vi "new FGGA Serial Data Server & Recordingv4.2.vi"(0 "VISA resource name out":refnum<visa-resource-name>, 11 "error IO":errorcluster) -> ()   [LabVIEW 2014]
uses:
  <vilib>/Platform/TimedLoop/XDataNode/timing_clust.ctl
  <vilib>/Platform/TimedLoop/XDataNode/nitl_modes.ctl
  <vilib>/Platform/TimedLoop/XDataNode/wakeup.ctl
  C:/Program Files (x86)/National Instruments/LabVIEW 2014/examples/Data Communication/Network Streams/Simple Network Streams/support/Network Stream Command.ctl
  <vilib>/Utility/error.llb/whitespace.ctl
  <vilib>/Instr/_visa.llb/VISA Configure Serial Port (Instr).vi
  <vilib>/Utility/tcp.llb/UDP Multicast Write-Only Open.vi
  <vilib>/platform/TimedLoop/XDataNode/XDataNode.xnode
  <vilib>/Platform/TimedLoop/XDataNode/XDNodeRunTimeDep.lvlib
panel:
  out "Unix time":u32
  out "FGGA Pump":bool
  out "Flight Number":string
  out "Stop File Write":bool
  out "Default file name":string
  out "MFC":dbl[](array[numeric])
  out "FGGA restart":bool
  out "V4":bool
  out "V3":bool
  out "V2":bool
  out "V1":bool
  out "error out 2":errorcluster
  out "error out":errorcluster
  in  "MFC_1 SLPM set value":dbl
  out "Value Read":string
  out "status":bool
  in  "VISA resource name":refnum<visa-resource-name>="ASRL3::INSTR"
  in  "timeout (10sec) 2":u32=3000
  in  "Clear Display\nErrors":bool
  out "Data Processing":bool
  out "TCP Binary Packet":string
  out "UDP Time Stamp Offset":i32=1
  out "Data String":string
  out "UDP_ACSII_Out":string
  out "Serial error out":errorcluster
  out "SEPTIC TCP Error Out":errorcluster
  out "TCP packet\nSend To SEPTIC":bool
  out "FISH TCP Error Out":errorcluster
  out "TCP packet\nSend To FISH":bool
  out "UDP_Pack_num":u32
  out "UDP_Out Status":bool
  out "UDP_Out_Error Out":errorcluster
  out "Data Array":string[](array[string])
  out "RAW DATA":string
  in  "stop":bool
  out "Number of times \nRead time out":u32
  out "Loop count":i32
  # "Date"
  # "Time"
  # "CH4_wet_ppm"
  # "1"
  # "CO4_wet_ppm_sd"
  # "H2O_ppm"
  # "3"
  # "H2O_ppm_sd"
  # "CO2_wet_ppm"
  # "5"
  # "CO2_wet_ppm_sd"
  # "CH4_dry_ppm"
  # "CH4_dry_ppm_sd"
  # "CO2_dry_ppm"
  # "CO2_dry_ppm_sd"
  # "cell_pressure_torr"
  # "11"
  # "cell_pressure_torr_sd"
  # "13"
  # "cell_temp_degC"
  # "cell_temp_degC_sdev"
  # "ambient(bench)_temp_degC"
  # "15"
  # "ambient(bench)_temp_dedgC_sd"
  # "17"
  # "RDA_us"
  # "RDA_us_sd"
  # "RDB_us"
  # "19"
  # "RDB_us_sd"
  # "Fitflag"
  # "21"
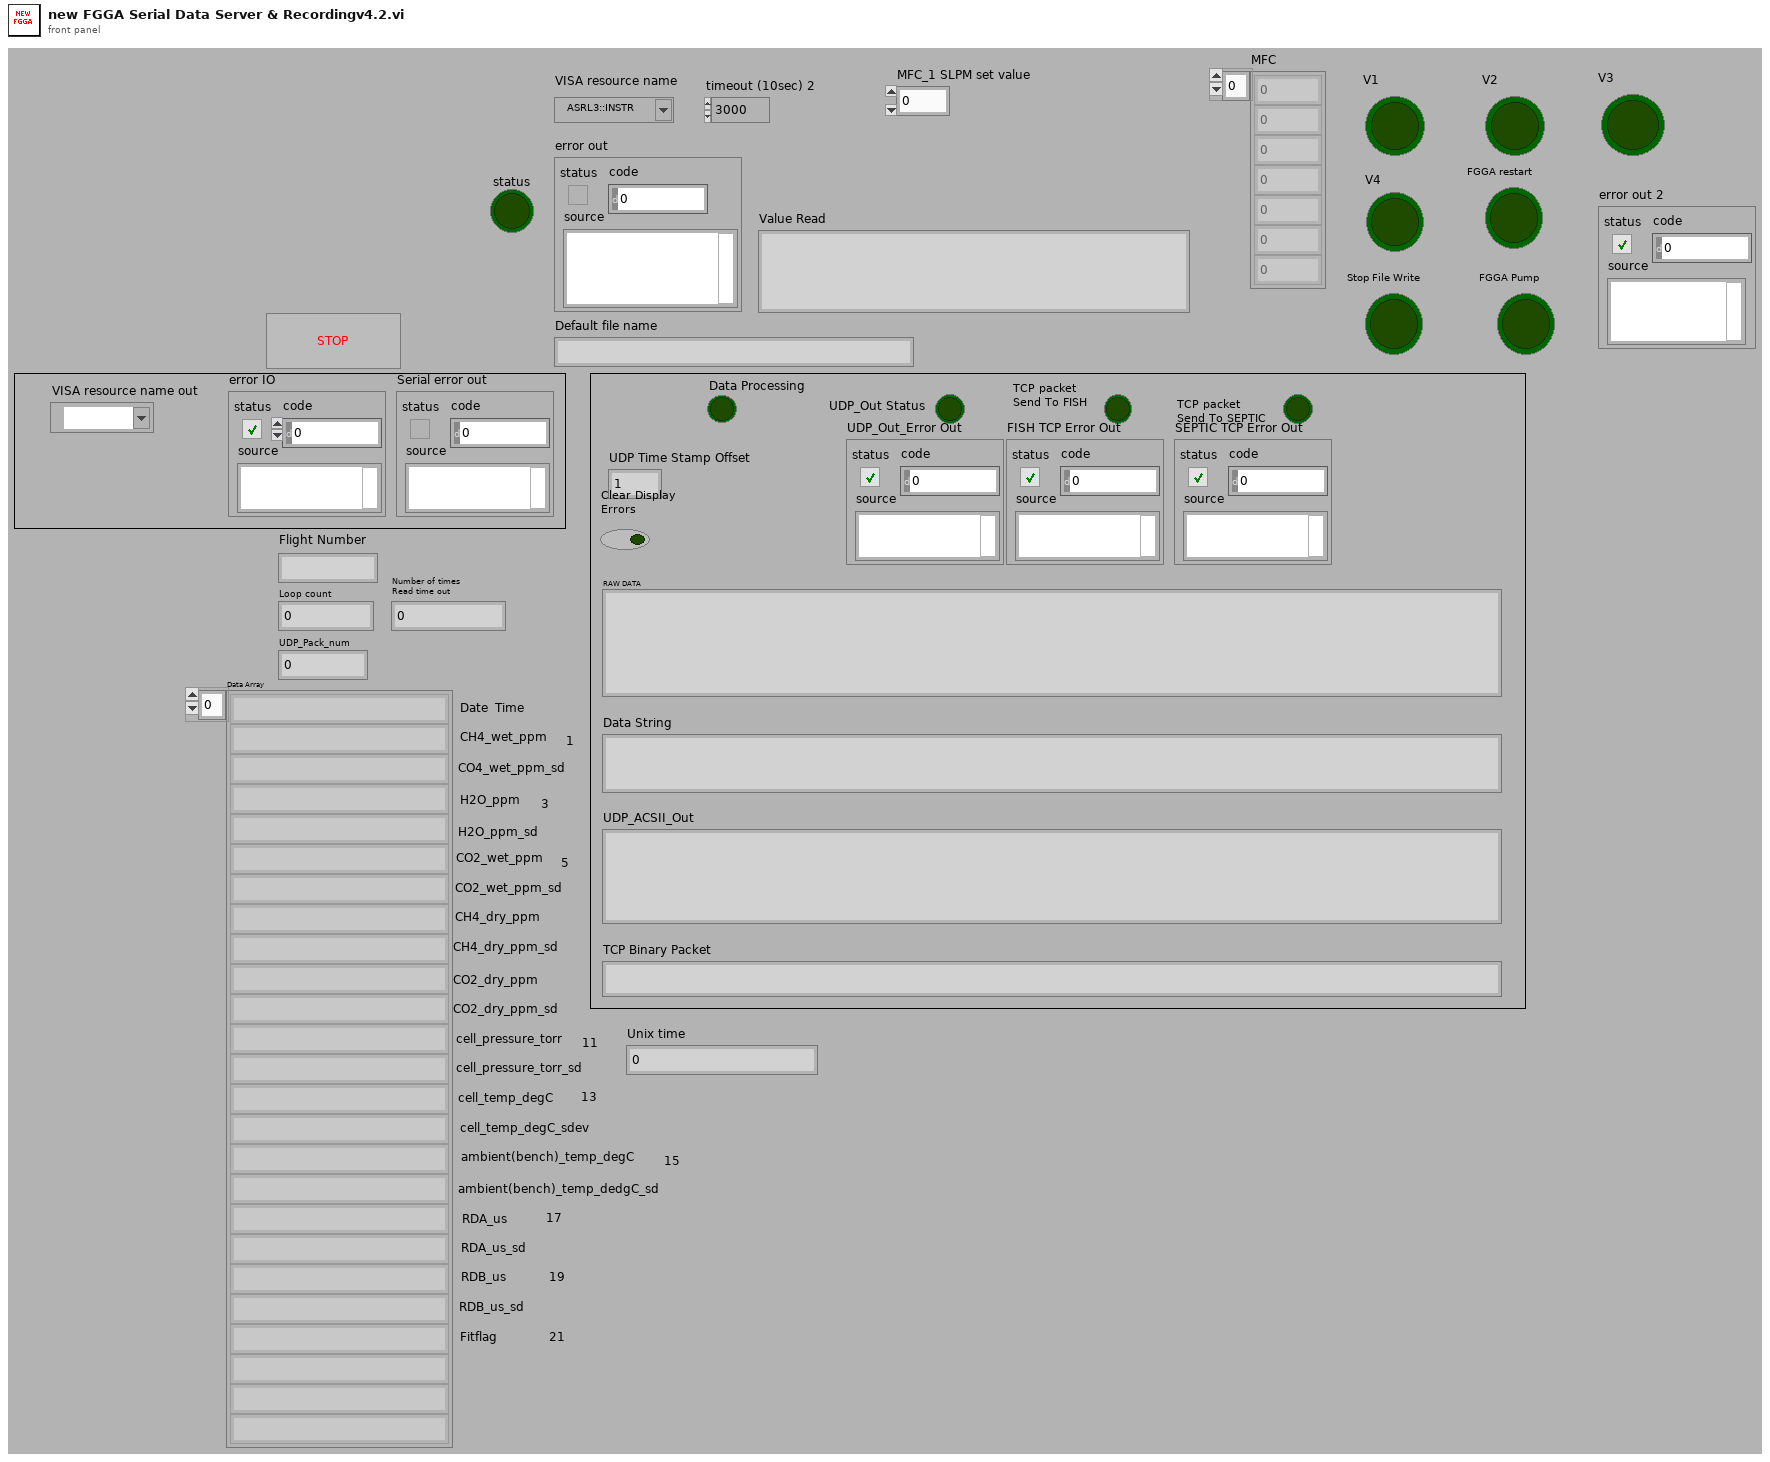
[diagram p1: front panel]
types:
  T1 = typedef "XDNodeRunTimeDep.lvlib/timing_clust.ctl" = cluster{"Expected End [f-1]":u64, "Actual End [f-1]":u64, "Finished Late? [f-1]":bool, "Expected End [i-1]":u64, "Actual End [i-1]":u64, "Finished Late? [i-1]":bool, "Expected Start [i]":u64, "Actual Start [i]":u64, "Expected Start [f]":u64, "Actual Start [f]":u64, "Source Name":string, "Structure Name":string, "Period":i64, "Deadline":i64, "Offset":i64, "Start":i64, "Priority":i32, "Timeout":i32, "Mode":T2, "Wakeup Reason":T3, "Error":errorcluster, "Source Type":string, "Secondary Source Type":string, "Global End Time":u64, "Global Start Time":u64, "Frame Duration":u64, "Iteration Duration":u64, "Assigned CPU":i32, "I/O Scan Engine Mode":u32}
  T2 = typedef "XDNodeRunTimeDep.lvlib/nitl_modes.ctl" = enum32{"No Change", "Process missed periods, maintain original phase", "Discard missed periods, maintain original phase", "Process missed periods, ignore original phase", "Discard missed periods, ignore original phase"}
  T3 = typedef "XDNodeRunTimeDep.lvlib/wakeup.ctl" = enum32{"Normal", "Aborted", "Asynchronous wakeup", "Timing source error", "Timed loop error", "Timeout"}
  T4 = enum16{"open", "replace", "create", "open or create", "replace or create", "replace or create with confirmation"}
  T5 = typedef "Network Stream Command.ctl" = cluster{"Message":string, "Message Data":variant}
  T6 = typedef "whitespace.ctl" = u16
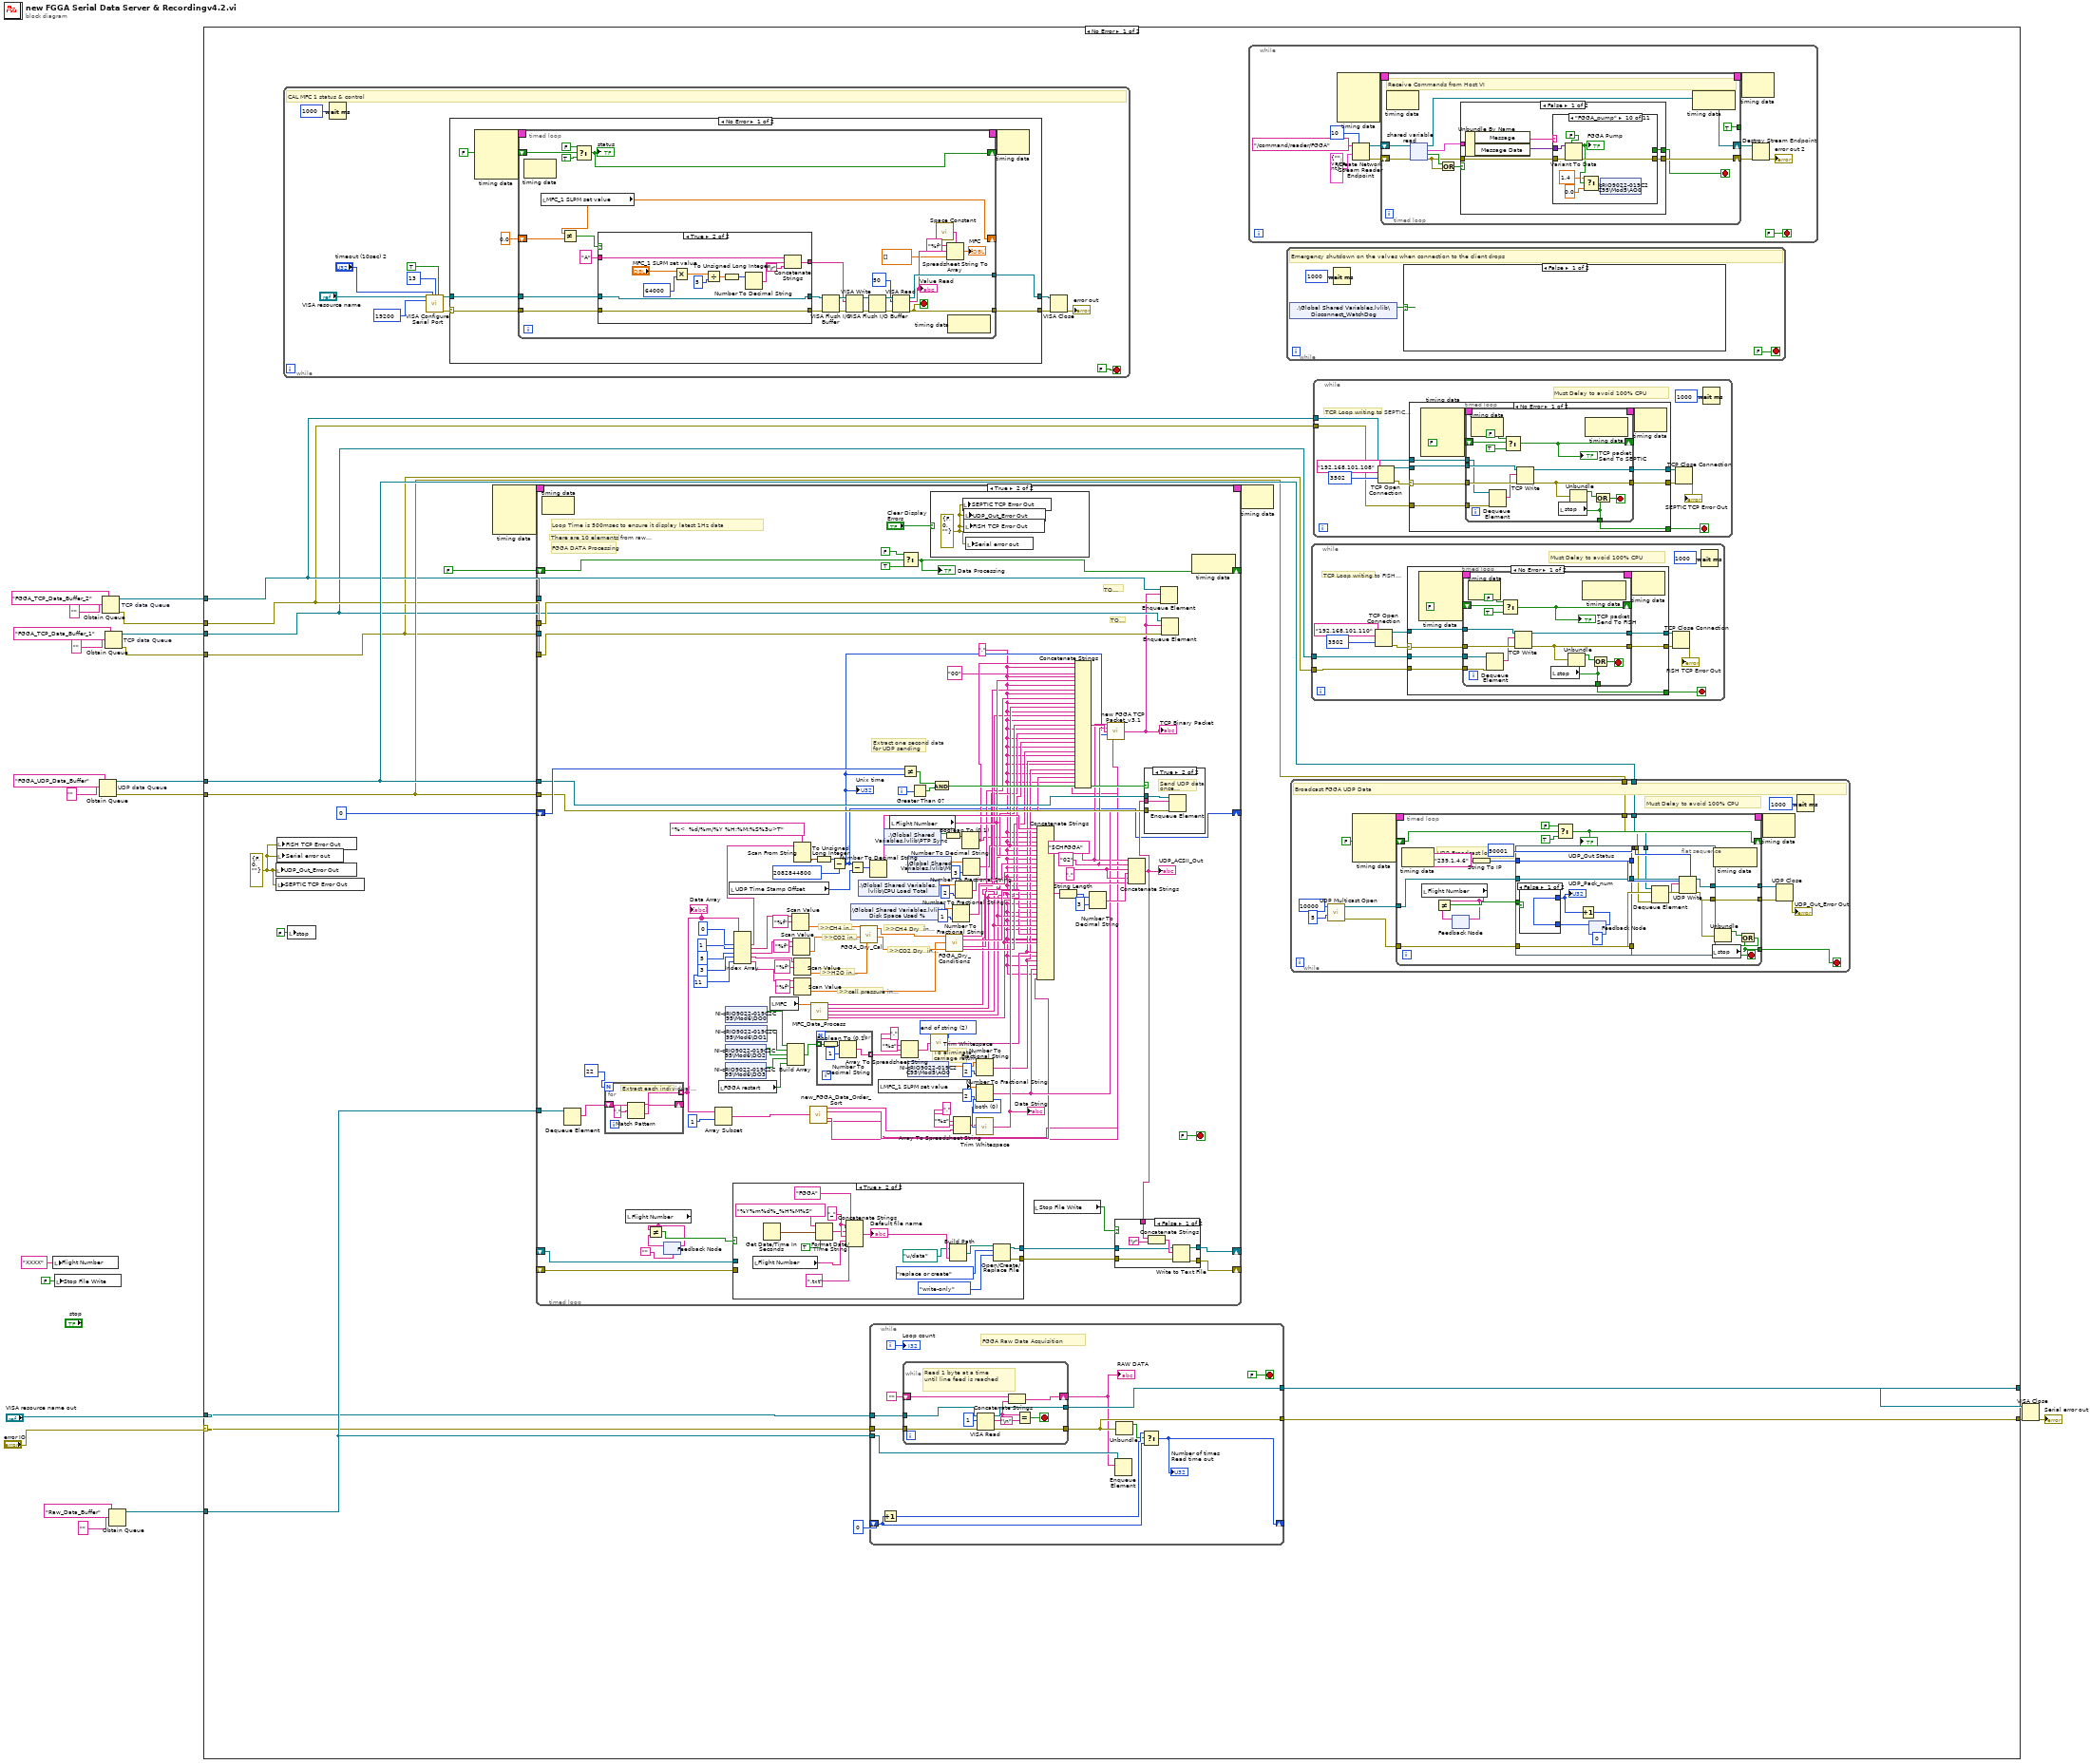
[diagram p0: block diagram]
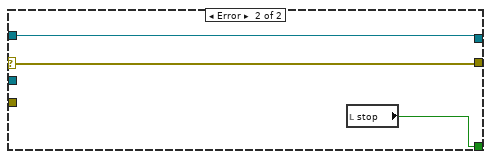
[diagram p2: hidden frame]
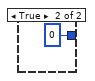
[diagram p3: hidden frame]
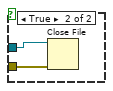
[diagram p5: hidden frame]
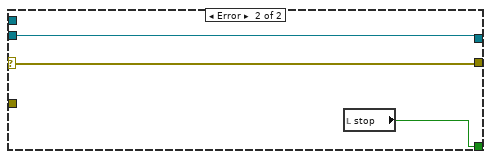
[diagram p8: hidden frame]
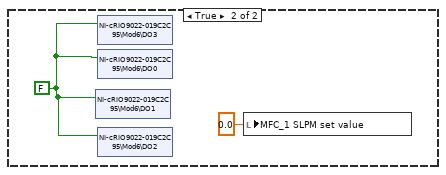
[diagram p9: hidden frame]
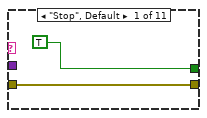
[diagram p10: hidden frame]
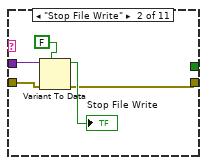
[diagram p11: hidden frame]
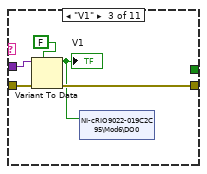
[diagram p12: hidden frame]
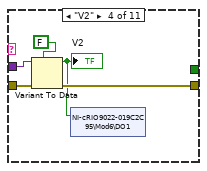
[diagram p13: hidden frame]
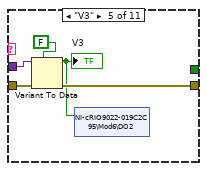
[diagram p14: hidden frame]
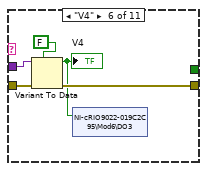
[diagram p15: hidden frame]
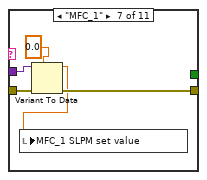
[diagram p16: hidden frame]
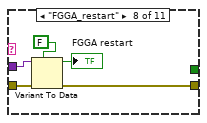
[diagram p17: hidden frame]
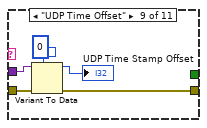
[diagram p18: hidden frame]
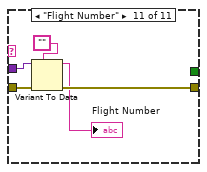
[diagram p19: hidden frame]
diagram:
  n1 = local write "Flight Number"("XXXX" ("Flight Number")) -> ()
  n2 = local write "Stop File Write"(FALSE ("Stop File Write")) -> ()
  n3 = Obtain Queue "UDP data Queue"(name (unnamed)="FGGA_UDP_Data_Buffer", element data type="") -> (queue out=w14:refnum<queue>, error out=w13:errorcluster)  [unwired: 3 in, 1 out]
  n4 = Obtain Queue "TCP data Queue"(name (unnamed)="FGGA_TCP_Data_Buffer_2", element data type="") -> (queue out=w8:refnum<queue>, error out=w7:errorcluster)  [unwired: 3 in, 1 out]
  n5 = Obtain Queue "TCP data Queue"(name (unnamed)="FGGA_TCP_Data_Buffer_1", element data type="") -> (queue out=w6:refnum<queue>, error out=w5:errorcluster)  [unwired: 3 in, 1 out]
  n6 = Obtain Queue(name (unnamed)="Raw_Data_Buffer", element data type="") -> (queue out=w20:refnum<queue>)  [unwired: 3 in, 2 out]
  n7 = case shown="No Error" "error IO" {
    selector: "error IO" -> [w27 w536]
    tunnel: "VISA resource name out" -> [w28 w537]
    tunnel: [w39 w537] -> w17
    tunnel: [w40 w536] -> w18
    tunnel: w20 -> [w38 _]
    tunnel: w14 -> [w36 _]
    tunnel: w13 -> [w35 _]
    tunnel: w8 -> [w34 _]
    tunnel: w7 -> [w33 _]
    tunnel: w6 -> [w32 _]
    tunnel: w5 -> [w31 _]
    frame No Error {
      w23 = errorcluster {"status"=FALSE, "code"=0, "source"=""} ("UDP Error Out")
      n8 = local write "UDP_Out_Error Out"(w23) -> ()
      n9 = local write "SEPTIC TCP Error Out"(w23) -> ()
      n10 = local write "FISH TCP Error Out"(w23) -> ()
      n11 = local write "Serial error out"(w23) -> ()
      n12 = while {
        stop <- FALSE stop-if-true
        # "CAL MFC 1 status & control"
        n13 = Wait (ms)(milliseconds to wait=u32 1000) -> ()  [unwired: 1 out]
        n14 = call-poly "VISA Configure Serial Port"("VISA resource name"="VISA resource name", "timeout (10sec)"="timeout (10sec) 2", "termination char\n(0xA = '\\n' = LF)"=u8 13 ("termination char\n(0xA = '\\n' = LF)"), "Enable Termination\nChar (T)"=TRUE ("Enable Termination\nChar (T)"), "baud rate (9600)"=u32 19200) -> ("VISA resource name out"=w477:refnum<visa-resource-name>, "error out"=w473:errorcluster)  [unwired: 9 in]
        n15 = case shown="No Error" w473 {
          selector: w473 -> [w484 w534]
          tunnel: w477 -> [w485 w535]
          tunnel: [w483 w535] -> w476
          tunnel: [w482 w534] -> w475
          frame No Error {
            n16 = node-c288() -> (w480:T1)  [unwired: 4 in]
            n17 = timed-loop {
              tunnel: w485 -> [w508]
              tunnel: w484 -> [w506]
              tunnel: [w499] -> w483
              tunnel: [w494] -> w482
              shift-right: [w495] -> _
              shift-left: FALSE -> [w498]
              timing: w480 -> [_]
              timing-out: [_] -> w479
              shift-right: [w486] -> _
              shift-left: 0.0 -> [w488]
              stop <- w494 stop-if-true
              n18 = node-c288() -> ()  [unwired: 1 in, 1 out]
              n19 = local read "MFC_1 SLPM set value"() -> (w486:dbl)
              n20 = Not Equal?(x=w486, y=w488) -> (x != y?=w487:bool)
              n21 = Select(t=FALSE, s=w498, f=TRUE) -> (s? t:f=w495:bool)
              "status" <- w495
              n22 = case shown="True" w487 {
                tunnel: w508 -> [w516 w531]
                tunnel: [w516 w531] -> w507
                tunnel: w506 -> [w515 w530]
                tunnel: [w515 w530] -> w505
                tunnel: "A" -> [w519 w523]
                tunnel: [w517 w520] -> w503
                frame False {
                  n23 = Concatenate Strings(w519, "\r") -> (w517:string)
                }
                frame True {
                  n24 = Multiply(x="MFC_1 SLPM set value", y=u32 64000) -> (x*y=w527:dbl)
                  n25 = Divide(x=w527, y=u32 5) -> (x/y=w525:dbl)
                  n26 = To Unsigned Long Integer(number=w525) -> (unsigned 32bit integer=w524:u32)
                  n27 = Number To Decimal String(number=w524) -> (decimal integer string=w522:string)  [unwired: 1 in]
                  n28 = Concatenate Strings(w523, w522, "\r") -> (w520:string)
                }
              }
              n29 = VISA Flush I/O Buffer(VISA resource name=w507, error in (no error)=w505) -> (VISA resource name out=w510:refnum<visa-resource-name>, error out=w509:errorcluster)  [unwired: 1 in]
              n30 = VISA Write(VISA resource name=w510, write buffer=w503, error in (no error)=w509) -> (VISA resource name out=w502:refnum<visa-resource-name>, error out=w501:errorcluster)  [unwired: 1 out]
              n31 = VISA Flush I/O Buffer(VISA resource name=w502, error in (no error)=w501) -> (VISA resource name out=w512:refnum<visa-resource-name>, error out=w511:errorcluster)  [unwired: 1 in]
              n32 = VISA Read(VISA resource name=w512, byte count=u32 50, error in (no error)=w511) -> (VISA resource name out=w499:refnum<visa-resource-name>, read buffer=w493:string, error out=w494:errorcluster)  [unwired: 1 out]
              "Value Read" <- w493
              n33 = call <vilib>:"Space Constant.vi"() -> ("String"=w492:string)
              n34 = Spreadsheet String To Array(delimiter (Tab)=w492, format string="%f", spreadsheet string=w493, array type (2D Dbl)=dbl[] []) -> (array=→"MFC":dbl[])
              n35 = node-c288() -> ()  [unwired: 1 in, 1 out]
            }
            n36 = node-c288(w479) -> ()  [unwired: 1 out]
          }
          frame Error {
          }
        }
        n37 = VISA Close(VISA resource name=w476, error in (no error)=w475) -> (error out=→"error out":errorcluster)
      }
      n38 = local write "stop"(FALSE ("stop")) -> ()
      n39 = node-c288() -> (w25:T1)  [unwired: 4 in]
      n40 = timed-loop {
        timing: w25 -> [_]
        timing-out: [_] -> w24
        tunnel: w38 -> [w265]
        tunnel: w36 -> [w230]
        tunnel: w35 -> [w229]
        shift-right: [w155] -> _
        shift-left: u32 0 -> [w233]
        tunnel: w34 -> [w228]
        tunnel: w33 -> [w227]
        tunnel: w32 -> [w226]
        tunnel: w31 -> [w225]
        shift-right: [w221] -> _
        shift-left: FALSE -> [w224]
        shift-right: [w210] -> _
        shift-left: _ -> [w202]
        shift-right: [w200] -> _
        shift-left: _ -> [w201]
        i -> [w232]
        stop <- FALSE stop-if-true
        w174 = T6 2 items=["both", "start of string", "end of string"] ("location (both)")
        w148 = ","
        w251 = T6 0 items=["both", "start of string", "end of string"] ("location (both)")
        w259 = ","
        w156 = "02"
        w157 = "$CHFGGA"
        # "To eliminate\ncarriage return"
        # ">>cell pressure in torr>>"
        # "There are 10 elements from raw packet"
        # "TO SEPTIC"
        # "TO FISH"
        # "Extract one second data\nfor UDP sending"
        # ">>CO2 Dry  in ppm>>"
        # ">>CH4 Dry  in ppb>>"
        # ">>H2O in ppm>>"
        # ">>CO2 in ppm>>"
        # ">>CH4 in ppm>>"
        # "Loop Time is 500msec to ensure it display latest 1Hz data"
        # "FGGA DATA Processing"
        n41 = node-c288() -> ()  [unwired: 1 in, 1 out]
        n42 = Dequeue Element(queue=w265) -> (element=w220:string)  [unwired: 2 in, 3 out]
        n43 = for {
          N: 22 -> [_]
          shift-right: [w302] -> _
          shift-left: w220 -> [w300]
          tunnel: [w301] -> w256 mode=indexing
          # "Extract each individual param"
          n44 = Match Pattern(string=w300, regular expression=",") -> (before substring=w301:string, after substring=w302:string)  [unwired: 1 in, 2 out]
        }
        "Data Array" <- w256
        n45 = local read "Flight Number"() -> (w199:string)
        n46 = feedback #1("" ("Flight Number")) -> (w207:string)
        n47 = Not Equal?(x=w199, y=w207) -> (x != y?=w205:bool)
        n48 = feedback-in #1(w199) -> ()
        n49 = Array Subset(array=w256, index=1) -> (w146:string[])  [unwired: 1 in]
        n50 = local read "FGGA restart"() -> (w184:bool)
        n51 = shared-variable "NI-cRIO9022-019C2C95\\Mod6\\DO2"() -> (w190:bool)  [unwired: 1 in, 1 out]
        n52 = shared-variable "NI-cRIO9022-019C2C95\\Mod6\\DO3"() -> (w189:bool)  [unwired: 1 in, 1 out]
        n53 = shared-variable "NI-cRIO9022-019C2C95\\Mod6\\DO0"() -> (w192:bool)  [unwired: 1 in, 1 out]
        n54 = shared-variable "NI-cRIO9022-019C2C95\\Mod6\\DO1"() -> (w191:bool)  [unwired: 1 in, 1 out]
        n55 = local read "UDP Time Stamp Offset"() -> (w173:i32)
        n56 = case shown="True" w205 {
          tunnel: [w271 w273] -> w204
          tunnel: [w270 w272] -> w203
          tunnel: w202 -> [w271 _]
          tunnel: w201 -> [w270 _]
          frame False {
          }
          frame True {
            w279 = "_" ("string")
            n57 = local read "Flight Number"() -> (w286:string)
            n58 = Get Date/Time In Seconds() -> (seconds since 1Jan1904=w274:timestamp)
            n59 = Format Date/Time String(time format string (%c)="%Y%m%d%_%H%M%S", seconds (now)=w274, UTC format=TRUE) -> (date/time string=w276:string)
            n60 = Concatenate Strings("FGGA" ("string"), w279, w276, w279, w286, ".txt" ("string")) -> (w281:string)
            "Default file name" <- w281
            n61 = Build Path(base path=path "u:/data", name or relative path=w281) -> (appended path=w285:path)
            n62 = Open/Create/Replace File(file path (use dialog)=w285, operation (0:open)=T4."replace or create", access (0:read/write)=enum16{"read/write", "read-only", "write-only"}."write-only") -> (refnum out=w273:refnum<file>, error out=w272:errorcluster)  [unwired: 3 in, 1 out]
          }
        }
        n63 = Index Array(array=w256, index #1=0 ("index"), index #2=1 ("index"), index #3=5 ("index"), index #4=3 ("index"), index #5=11 ("index")) -> (element #1=w149:string, element #2=w154:string, element #3=w153:string, element #4=w152:string, element #5=w151:string)
        n64 = local read "MFC"() -> (w211:dbl[])
        n65 = Build Array(w192, w191, w190, w189, w184) -> (w188:bool[])
        n66 = Scan Value(string=w154, format string="%f") -> (value=w242:dbl)  [unwired: 1 in, 1 out]
        n67 = Scan Value(string=w153, format string="%f") -> (value=w241:dbl)  [unwired: 1 in, 1 out]
        n68 = Scan From String(format string="%<  %d/%m/%Y %H:%M:%S%3u>T", input string=w149) -> (output 1=w238:timestamp)  [unwired: 3 in, 3 out]
        n69 = Scan Value(string=w152, format string="%f") -> (value=w212:dbl)  [unwired: 1 in, 1 out]
        n70 = Scan Value(string=w151, format string="%f") -> (value=w213:dbl)  [unwired: 1 in, 1 out]
        n71 = call "new_FGGA_Data_Order_Sort.vi"("Data In"=w146) -> ("UDP Data Out"=w145:string[], "UDP Ambient(bench)_temp"=w144:string, "TCP Data Out"=w143:string[], "TCP Ambient(bench)_temp"=w142:string)  [unwired: 11 in]
        n72 = call "MFC_Data_Process.vi"("MFC"=w211) -> ("MFC Absolute Pressure"=w168:string, "MFC Temperature"=w167:string, "MFC Volumetric Flow"=w166:string, "MFC Mass Flow"=w165:string, "MFC Set Point"=w164:string)  [unwired: 10 in]
        n73 = To Unsigned Long Integer(number=w238) -> (unsigned 32bit integer=w239:u32)
        n74 = for {
          tunnel: w188 -> [w268] mode=indexing
          tunnel: [w267] -> w185 mode=indexing
          n75 = Boolean To (0,1)(Boolean=w268) -> (0, 1=w269:i16)
          n76 = Number To Decimal String(number=w269, width (-)=i16 1) -> (decimal integer string=w267:string)
        }
        n77 = Subtract(x=w239, y=u32 2082844800) -> (x-y=w155:u32)
        "Unix time" <- w155
        n78 = Subtract(x=w155, y=w173) -> (x-y=w236:u32)
        n79 = shared-variable ".\\Global Shared Variables.lvlib\\Disk Space Used %"() -> (w177:dbl)  [unwired: 1 in, 1 out]
        n80 = shared-variable ".\\Global Shared Variables.lvlib\\CPU Load Total"() -> (w198:dbl)  [unwired: 1 in, 1 out]
        n81 = call "FGGA_Dry_Cal.vi"("H2O"=w212, "CO2_Wet"=w241, "CH4_Wet"=w242) -> ("CO2_Dry"=w215:dbl, "CH4_Dry"=w217:dbl)  [unwired: 7 in]
        n82 = Number To Decimal String(number=w236) -> (decimal integer string=w237:string)  [unwired: 1 in]
        n83 = local read "MFC_1 SLPM set value"() -> (w180:dbl)
        n84 = shared-variable ".\\Global Shared Variables.lvlib\\PTP Sync"() -> (w193:bool)  [unwired: 1 in, 1 out]
        n85 = local read "Flight Number"() -> (w172:string)
        n86 = Array To Spreadsheet String(delimiter (Tab)=",", array=w185, 3:"%s" ("format string")) -> (spreadsheet string=w175:string)
        n87 = Select(t=FALSE, s=w224, f=TRUE) -> (s? t:f=w221:bool)
        "Data Processing" <- w221
        n88 = Not Equal?(x=w233, y=w155) -> (x != y?=w234:bool)
        n89 = shared-variable ".\\Global Shared Variables.lvlib\\MFM"() -> (w196:dbl)  [unwired: 1 in, 1 out]
        n90 = shared-variable "NI-cRIO9022-019C2C95\\Mod5\\AO0"() -> (w182:dbl)  [unwired: 1 in, 1 out]
        n91 = Greater Than 0?(x=w232) -> (x > 0?=w235:bool)
        n92 = case shown="True" "Clear Display\nErrors" {
          frame False {
          }
          frame True {
            w296 = errorcluster {"status"=FALSE, "code"=0, "source"=""} ("UDP Error Out")
            n93 = local write "SEPTIC TCP Error Out"(w296) -> ()
            n94 = local write "UDP_Out_Error Out"(w296) -> ()
            n95 = local write "FISH TCP Error Out"(w296) -> ()
            n96 = local write "Serial error out"(w296) -> ()
          }
        }
        n97 = call <vilib>:"Trim Whitespace.vi"("string"=w175, "location (both)"=w174) -> ("trimmed string"=w163:string)
        n98 = Compound Arithmetic op=AND(w234, w235) -> (w231:bool)
        n99 = Boolean To (0,1)(Boolean=w193) -> (0, 1=w194:i16)
        n100 = call "FGGA_Dry_Conditions.vi"("CH4_Dry"=w217, "Pressure"=w213, "CO2_Dry"=w215) -> ("CH4_Dry_TCP"=w171:string, "CH4_Dry_UDP"=w219:string, "CO2_Dry_TCP"=w170:string, "CO2_Dry_UDP"=w218:string)  [unwired: 9 in]
        n101 = Number To Fractional String(number=w177, precision (6)=i16 1) -> (F-format string=w176:string)  [unwired: 2 in]
        n102 = Array To Spreadsheet String(delimiter (Tab)=",", array=w145, 3:"%s" ("format string")) -> (spreadsheet string=w250:string)
        n103 = Number To Fractional String(number=w198, precision (6)=i16 2) -> (F-format string=w179:string)  [unwired: 2 in]
        n104 = Number To Decimal String(number=w194) -> (decimal integer string=w159:string)  [unwired: 1 in]
        n105 = Number To Fractional String(number=w196, precision (6)=i16 3) -> (F-format string=w169:string)  [unwired: 2 in]
        n106 = Number To Fractional String(number=w182, precision (6)=i16 2) -> (F-format string=w162:string)  [unwired: 2 in]
        n107 = Number To Fractional String(number=w180, precision (6)=i16 2) -> (F-format string=w161:string)  [unwired: 2 in]
        n108 = call <vilib>:"Trim Whitespace.vi"("string"=w250, "location (both)"=w251) -> ("trimmed string"=w249:string)
        "Data String" <- w249
        n109 = local read "Stop File Write"() -> (w208:bool)
        n110 = Concatenate Strings(w237, w148, w159, w148, w169, w148, w172, w148, w179, w148, w176, w148, w249, w148, w219, w148, w218, w148, w168, w148, w167, w148, w166, w148, w165, w148, w164, w148, w163, w148, w162, w148, w161, w148, w144) -> (w258:string)
        n111 = String Length(string=w258) -> (length=w262:i32)
        n112 = Concatenate Strings(w159, w148, "00", w148, w172, w148, w171, w148, w170, w148, w169, w148, w168, w148, w167, w148, w166, w148, w165, w148, w164, w148, w163, w148, w162, w148, w161, w148, w142) -> (w160:string)
        n113 = Number To Decimal String(number=w262, width (-)=i16 3) -> (decimal integer string=w260:string)
        n114 = call "new FGGA TCP Packet_v3.1.vi"("ID"=w157, "Version"=w156, "TCP Packet In"=w160, "utc_time"=w155, "Data Array"=w143) -> ("TCP Binary Packet"=w147:string)  [unwired: 10 in]
        "TCP Binary Packet" <- w147
        n115 = Concatenate Strings(w157, w156, w259, w260, w259, w258) -> (w209:string)
        "UDP_ACSII_Out" <- w209
        n116 = case shown="False" w208 {
          tunnel: w209 -> [w293 _]
          tunnel: [w290 _] -> w210
          tunnel: w204 -> [w289 w295]
          tunnel: w203 -> [w288 w294]
          tunnel: [w287 _] -> w200
          frame False {
            n117 = Concatenate Strings(w293, "\r") -> (w291:string)
            n118 = Write to Text File(file (use dialog)=w289, text=w291, error in=w288) -> (refnum out=w290:refnum<file>, error out=w287:errorcluster)  [unwired: 2 out]
          }
          frame True {
            n119 = Close File(refnum=w295, error in=w294) -> ()  [unwired: 2 out]
          }
        }
        n120 = case shown="True" w231 {
          tunnel: w209 -> [_ w299]
          tunnel: w230 -> [_ w298]
          tunnel: w229 -> [_ w297]
          frame False {
          }
          frame True {
            # "Send UDP data once\na second"
            n121 = Enqueue Element(queue=w298, element=w299, error in (no error)=w297) -> ()  [unwired: 1 in, 3 out]
          }
        }
        n122 = Enqueue Element(queue=w228, element=w147, error in (no error)=w227) -> ()  [unwired: 1 in, 3 out]
        n123 = Enqueue Element(queue=w226, element=w147, error in (no error)=w225) -> ()  [unwired: 1 in, 3 out]
        n124 = node-c288() -> ()  [unwired: 1 in, 1 out]
      }
      n125 = while {
        tunnel: w28 -> [w362]
        tunnel: w27 -> [w361]
        tunnel: [w360] -> w40
        shift-right: [w356] -> _
        shift-left: u32 0 -> [w357]
        tunnel: [w359] -> w39
        tunnel: w38 -> [w353]
        i -> [w358]
        stop <- FALSE stop-if-true
        # "FGGA Raw Data Acquisition"
        n126 = Increment(x=w357) -> (x+1=w355:u32)
        n127 = while {
          tunnel: [w372] -> w359
          tunnel: [w371] -> w360
          tunnel: w362 -> [w370]
          tunnel: w361 -> [w369]
          shift-right: [w367] -> w352
          shift-left: "" -> [w368]
          stop <- w364 stop-if-true
          # "Read 1 byte at a time \nuntil line feed is reached"
          n128 = VISA Read(VISA resource name=w370, byte count=u32 1, error in (no error)=w369) -> (VISA resource name out=w372:refnum<visa-resource-name>, read buffer=w366:string, error out=w371:errorcluster)  [unwired: 1 out]
          n129 = Concatenate Strings(w368, w366) -> (w367:string)
          n130 = Equal?(x=w366, y="\n") -> (x = y?=w364:bool)
        }
        "RAW DATA" <- w352
        n131 = Enqueue Element(queue=w353, element=w352) -> ()  [unwired: 2 in, 3 out]
        n132 = Unbundle(w360) -> ("status"=w351:bool)  [unwired: 2 out]
        n133 = Select(t=w355, s=w351, f=w357) -> (s? t:f=w356:u32)
        "Number of times \nRead time out" <- w356
        "Loop count" <- w358
      }
      n134 = node-c288(w24) -> ()  [unwired: 1 out]
      n135 = while {
        stop <- FALSE stop-if-true
        n136 = node-c288() -> (w379:T1)  [unwired: 4 in]
        n137 = Create Network Stream Reader Endpoint(7:10 ("reader buffer size"), 9:T5 {"Message"="", "Message Data"=variant} ("Message Cluster"), 11:"/command/reader/FGGA" ("reader url")) -> (0:w384:errorcluster, 3:w385:refnum<k21>)  [unwired: 4 in]
        n138 = timed-loop "Host->Target Command Reader" {
          shift-right: [w395] -> w382
          shift-left: w384 -> [w398]
          shift-right: [w396] -> w381
          shift-left: w385 -> [w397]
          tunnel: [TRUE] -> _
          timing: w379 -> [_]
          timing-out: [_] -> w378
          stop <- w389 stop-if-true
          # "Receive Commands from Host VI"
          n139 = node-c288() -> ()  [unwired: 1 in, 1 out]
          n140 = shared-variable-read(w397, w398) -> (w396:refnum<k21>, w391:errorcluster, w393:bool, w394:T5)  [unwired: 1 in]
          n141 = Or(x=w393, y=w391) -> (x .or. y?=w392:bool)
          n142 = case shown="False" w392 {
            selector: w392 -> [_ w462]
            tunnel: w391 -> [w406 w463]
            tunnel: [w405 w463] -> w395
            tunnel: w394 -> [w403 _]
            tunnel: [w404 w462] -> w389
            frame False {
              n143 = Unbundle By Name(w403) -> ("Message"=w402:string, "Message Data"=w401:variant)
              n144 = case shown="\"FGGA_pump\"" w402 {
                tunnel: w406 -> [w408 w413 w418 w423 w428 w433 w438 w443 w448 w456 w461]
                tunnel: [w408 w409 w417 w422 w427 w432 w437 w442 w447 w455 w460] -> w405
                tunnel: w401 -> [_ w412 w416 w421 w426 w431 w436 w441 w446 w454 w459]
                tunnel: [TRUE _ _ _ _ _ _ _ _ _ _] -> w404
                frame "Stop", Default {
                }
                frame "Stop File Write" {
                  n145 = Variant To Data(error in=w413, type=FALSE, Variant=w412) -> (data=→"Stop File Write":bool, error out=w409:errorcluster)
                }
                frame "V1" {
                  n146 = Variant To Data(error in=w418, type=FALSE, Variant=w416) -> (data=w414:bool, error out=w417:errorcluster)
                  "V1" <- w414
                  n147 = shared-variable "NI-cRIO9022-019C2C95\\Mod6\\DO0"(w414) -> ()  [unwired: 1 in, 1 out]
                }
                frame "V2" {
                  n148 = Variant To Data(error in=w423, type=FALSE, Variant=w421) -> (data=w419:bool, error out=w422:errorcluster)
                  "V2" <- w419
                  n149 = shared-variable "NI-cRIO9022-019C2C95\\Mod6\\DO1"(w419) -> ()  [unwired: 1 in, 1 out]
                }
                frame "V3" {
                  n150 = Variant To Data(error in=w428, type=FALSE, Variant=w426) -> (data=w424:bool, error out=w427:errorcluster)
                  "V3" <- w424
                  n151 = shared-variable "NI-cRIO9022-019C2C95\\Mod6\\DO2"(w424) -> ()  [unwired: 1 in, 1 out]
                }
                frame "V4" {
                  n152 = Variant To Data(error in=w433, type=FALSE, Variant=w431) -> (data=w429:bool, error out=w432:errorcluster)
                  "V4" <- w429
                  n153 = shared-variable "NI-cRIO9022-019C2C95\\Mod6\\DO3"(w429) -> ()  [unwired: 1 in, 1 out]
                }
                frame "MFC_1" {
                  n154 = Variant To Data(error in=w438, type=0.0, Variant=w436) -> (data=w434:dbl, error out=w437:errorcluster)
                  n155 = local write "MFC_1 SLPM set value"(w434) -> ()
                }
                frame "FGGA_restart" {
                  n156 = Variant To Data(error in=w443, type=FALSE, Variant=w441) -> (data=→"FGGA restart":bool, error out=w442:errorcluster)
                }
                frame "UDP Time Offset" {
                  n157 = Variant To Data(error in=w448, type=0, Variant=w446) -> (data=→"UDP Time Stamp Offset":i32, error out=w447:errorcluster)
                }
                frame "FGGA_pump" {
                  n158 = Variant To Data(error in=w456, type=FALSE, Variant=w454) -> (data=w451:bool, error out=w455:errorcluster)
                  "FGGA Pump" <- w451
                  n159 = Select(t=1.4 ("f"), s=w451, f=0.0 ("t")) -> (s? t:f=w452:dbl)
                  n160 = shared-variable "NI-cRIO9022-019C2C95\\Mod5\\AO0"(w452) -> ()  [unwired: 1 in, 1 out]
                }
                frame "Flight Number" {
                  n161 = Variant To Data(error in=w461, type="", Variant=w459) -> (data=→"Flight Number":string, error out=w460:errorcluster)
                }
              }
            }
            frame True {
            }
          }
          n162 = node-c288() -> ()  [unwired: 1 in, 1 out]
        }
        n163 = node-c288(w378) -> ()  [unwired: 1 out]
        n164 = Destroy Stream Endpoint(8:w382, 11:w381) -> (0:→"error out 2":errorcluster)
      }
      n165 = while {
        stop <- FALSE stop-if-true
        # "Emergency shutdown on the valves when connection to the client drops"
        n166 = shared-variable ".\\Global Shared Variables.lvlib\\Disconnect_WatchDog"() -> (w373:bool)  [unwired: 1 in, 1 out]
        n167 = Wait (ms)(milliseconds to wait=u32 1000) -> ()  [unwired: 1 out]
        n168 = case shown="False" w373 {
          frame False {
          }
          frame True {
            w377 = FALSE
            n169 = shared-variable "NI-cRIO9022-019C2C95\\Mod6\\DO1"(w377) -> ()  [unwired: 1 in, 1 out]
            n170 = shared-variable "NI-cRIO9022-019C2C95\\Mod6\\DO3"(w377) -> ()  [unwired: 1 in, 1 out]
            n171 = shared-variable "NI-cRIO9022-019C2C95\\Mod6\\DO0"(w377) -> ()  [unwired: 1 in, 1 out]
            n172 = shared-variable "NI-cRIO9022-019C2C95\\Mod6\\DO2"(w377) -> ()  [unwired: 1 in, 1 out]
            n173 = local write "MFC_1 SLPM set value"(0.0 ("MFC_1 SLPM set value")) -> ()
          }
        }
      }
      n174 = while {
        tunnel: w36 -> [w85]
        tunnel: w35 -> [w84]
        stop <- w86 stop-if-true
        # "Must Delay to avoid 100% CPU"
        # "Broadcast FGGA UDP Data"
        n175 = call-poly <vilib>:"UDP Multicast Open.vi"("time-to-live (1)"=u16 5, "port"=u16 10000) -> ("error out"=w93:errorcluster, "connection ID"=w94:refnum<k16>)  [unwired: 8 in]
        n176 = node-c288() -> (w96:T1)  [unwired: 4 in]
        n177 = timed-loop {
          tunnel: w94 -> [w117]
          tunnel: w93 -> [w116]
          timing: w96 -> [_]
          timing-out: [_] -> w95
          shift-right: [w105] -> _
          shift-left: FALSE -> [w108]
          tunnel: [w104] -> w88
          tunnel: [w102] -> w87
          tunnel: [w100] -> w86
          tunnel: w85 -> [w98]
          tunnel: w84 -> [w97]
          stop <- w101 stop-if-true
          # "UDP Broadcast loop"
          n178 = node-c288() -> ()  [unwired: 1 in, 1 out]
          n179 = local read "Flight Number"() -> (w99:string)
          n180 = feedback-in #2(w99) -> ()
          n181 = feedback #2() -> (w110:string)  [unwired: 1 in]
          n182 = Not Equal?(x=w99, y=w110) -> (x != y?=w109:bool)
          n183 = String To IP(1:"239.1.4.6" ("name")) -> (0:w114:u32)
          n184 = flat-sequence {
            tunnel: w114 -> [w124]
            tunnel: w116 -> [w125]
            tunnel: w117 -> [w126]
            tunnel: [w126] -> w113
            tunnel: [w125] -> w112
            tunnel: [w124] -> w111
            tunnel: w109 -> [w123]
            tunnel: u16 50001 ("port or service name") -> [w137]
            tunnel: w113 -> [w136]
            tunnel: w112 -> [w135]
            tunnel: w111 -> [w134]
            tunnel: [w133] -> w104
            tunnel: [w132] -> w102
            tunnel: w98 -> [w130]
            tunnel: w97 -> [w129]
            frame #0 {
              n185 = feedback #3(u32 0) -> (w120:u32)
              n186 = case shown="False" w123 {
                tunnel: w120 -> [w127 _]
                tunnel: [w127 u32 0] -> w119
                frame False {
                }
                frame True {
                }
              }
              "UDP_Pack_num" <- w119
              n187 = Increment(x=w119) -> (x+1=w121:u32)
              n188 = feedback-in #3(w121) -> ()
            }
            frame #1 {
              n189 = Dequeue Element(queue=w130, error in (no error)=w129) -> (element=w131:string)  [unwired: 1 in, 3 out]
              n190 = UDP Write(address=w134, port or service name=w137, connection ID=w136, data in=w131, 8:w135) -> (error out=w132:errorcluster, 3:w133:refnum<k16>)  [unwired: 1 in]
            }
          }
          n191 = Select(t=FALSE, s=w108, f=TRUE) -> (s? t:f=w105:bool)
          "UDP_Out Status" <- w105
          n192 = local read "stop"() -> (w100:bool)
          n193 = node-c288() -> ()  [unwired: 1 in, 1 out]
          n194 = Unbundle(w102) -> ("status"=w103:bool)  [unwired: 2 out]
          n195 = Compound Arithmetic op=OR(w103, w100) -> (w101:bool)
        }
        n196 = node-c288(w95) -> ()  [unwired: 1 out]
        n197 = UDP Close(connection ID=w88, 8:w87) -> (error out=→"UDP_Out_Error Out":errorcluster)  [unwired: 1 out]
        n198 = Wait (ms)(milliseconds to wait=u32 1000) -> ()  [unwired: 1 out]
      }
      n199 = while {
        tunnel: w32 -> [w43]
        tunnel: w31 -> [w42]
        stop <- w46 stop-if-true
        # "Must Delay to avoid 100% CPU"
        # "TCP Loop writing to FISH Tank"
        n200 = TCP Open Connection(address="192.168.101.110", remote port or service name=u16 3502) -> (connection ID=w49:refnum<k5>, error out=w44:errorcluster)  [unwired: 3 in]
        n201 = case shown="No Error" w44 {
          selector: w44 -> [w54 w81]
          tunnel: w49 -> [w59 w82]
          tunnel: [w58 w82] -> w48
          tunnel: [w57 w81] -> w47
          tunnel: [w56 w80] -> w46
          tunnel: w43 -> [w53 _]
          tunnel: w42 -> [w52 _]
          frame No Error {
            n202 = node-c288() -> (w61:T1)  [unwired: 4 in]
            n203 = timed-loop {
              tunnel: w59 -> [w75]
              tunnel: w54 -> [w74]
              tunnel: [w73] -> w58
              tunnel: [w72] -> w57
              tunnel: [w64] -> w56
              shift-right: [w66] -> _
              shift-left: FALSE -> [w69]
              timing: w61 -> [_]
              timing-out: [_] -> w60
              tunnel: w53 -> [w63]
              tunnel: w52 -> [w62]
              stop <- w70 stop-if-true
              n204 = node-c288() -> ()  [unwired: 1 in, 1 out]
              n205 = Dequeue Element(queue=w63, error in (no error)=w62) -> (element=w65:string)  [unwired: 1 in, 3 out]
              n206 = Select(t=FALSE, s=w69, f=TRUE) -> (s? t:f=w66:bool)
              "TCP packet\nSend To FISH" <- w66
              n207 = TCP Write(connection ID=w75, data in=w65, error in (no error)=w74) -> (connection ID out=w73:refnum<k5>, error out=w72:errorcluster)  [unwired: 1 in, 1 out]
              n208 = local read "stop"() -> (w64:bool)
              n209 = Unbundle(w72) -> ("status"=w71:bool)  [unwired: 2 out]
              n210 = node-c288() -> ()  [unwired: 1 in, 1 out]
              n211 = Compound Arithmetic op=OR(w71, w64) -> (w70:bool)
            }
            n212 = node-c288(w60) -> ()  [unwired: 1 out]
          }
          frame Error {
            n213 = local read "stop"() -> (w80:bool)
          }
        }
        n214 = TCP Close Connection(connection ID=w48, error in (no error)=w47) -> (error out=→"FISH TCP Error Out":errorcluster)  [unwired: 1 in, 1 out]
        n215 = Wait (ms)(milliseconds to wait=u32 1000) -> ()  [unwired: 1 out]
      }
      n216 = while {
        tunnel: w34 -> [w310]
        tunnel: w33 -> [w309]
        stop <- w313 stop-if-true
        # "Must Delay to avoid 100% CPU"
        # "TCP Loop writing to SEPTIC Tank"
        n217 = TCP Open Connection(address="192.168.101.108", remote port or service name=u16 3502) -> (connection ID=w316:refnum<k5>, error out=w311:errorcluster)  [unwired: 3 in]
        n218 = case shown="No Error" w311 {
          selector: w311 -> [w321 w348]
          tunnel: w316 -> [w326 w349]
          tunnel: [w325 w349] -> w315
          tunnel: [w324 w348] -> w314
          tunnel: [w323 w347] -> w313
          tunnel: w310 -> [w320 _]
          tunnel: w309 -> [w319 _]
          frame No Error {
            n219 = node-c288() -> (w328:T1)  [unwired: 4 in]
            n220 = timed-loop {
              tunnel: w326 -> [w342]
              tunnel: w321 -> [w341]
              tunnel: [w340] -> w325
              tunnel: [w339] -> w324
              tunnel: [w331] -> w323
              shift-right: [w333] -> _
              shift-left: FALSE -> [w336]
              timing: w328 -> [_]
              timing-out: [_] -> w327
              tunnel: w320 -> [w330]
              tunnel: w319 -> [w329]
              stop <- w337 stop-if-true
              n221 = node-c288() -> ()  [unwired: 1 in, 1 out]
              n222 = Dequeue Element(queue=w330, error in (no error)=w329) -> (element=w332:string)  [unwired: 1 in, 3 out]
              n223 = Select(t=FALSE, s=w336, f=TRUE) -> (s? t:f=w333:bool)
              "TCP packet\nSend To SEPTIC" <- w333
              n224 = TCP Write(connection ID=w342, data in=w332, error in (no error)=w341) -> (connection ID out=w340:refnum<k5>, error out=w339:errorcluster)  [unwired: 1 in, 1 out]
              n225 = local read "stop"() -> (w331:bool)
              n226 = Unbundle(w339) -> ("status"=w338:bool)  [unwired: 2 out]
              n227 = node-c288() -> ()  [unwired: 1 in, 1 out]
              n228 = Compound Arithmetic op=OR(w338, w331) -> (w337:bool)
            }
            n229 = node-c288(w327) -> ()  [unwired: 1 out]
          }
          frame Error {
            n230 = local read "stop"() -> (w347:bool)
          }
        }
        n231 = TCP Close Connection(connection ID=w315, error in (no error)=w314) -> (error out=→"SEPTIC TCP Error Out":errorcluster)  [unwired: 1 in, 1 out]
        n232 = Wait (ms)(milliseconds to wait=u32 1000) -> ()  [unwired: 1 out]
      }
    }
    frame Error {
    }
  }
  n233 = VISA Close(VISA resource name=w17, error in (no error)=w18) -> (error out=→"Serial error out":errorcluster)
